vi "EventsDemo-Empty.vi"() -> ()   [LabVIEW 2014]
doc: "Use this template to build a user interface event handler design pattern. Use this pattern for dialog boxes and other user interfaces. You also can create and execute user-defined events that the VI can handle the same way as user interface events."
panel:
  in  "stop":bool
  out "Blink":bool
  in  "Blink Rate (ms)":i32
  in  "Value In":dbl(slide) scale=0.0..10.0
  out "Last Button":cluster{"1":bool, "2":bool, "3":bool}
  out "2 x Value":dbl
  in  "Button 3":bool
  in  "Button 2":bool
  in  "Button 1":bool
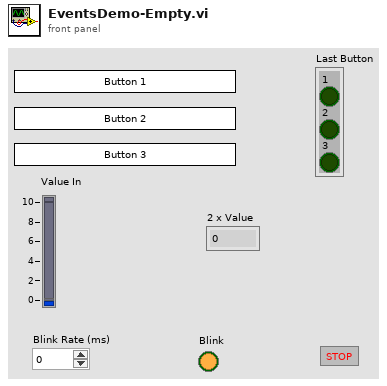
[diagram p1: front panel]
types:
  T1 = cluster{"Button 1":bool, "Button 2":bool, "Button 3":bool}
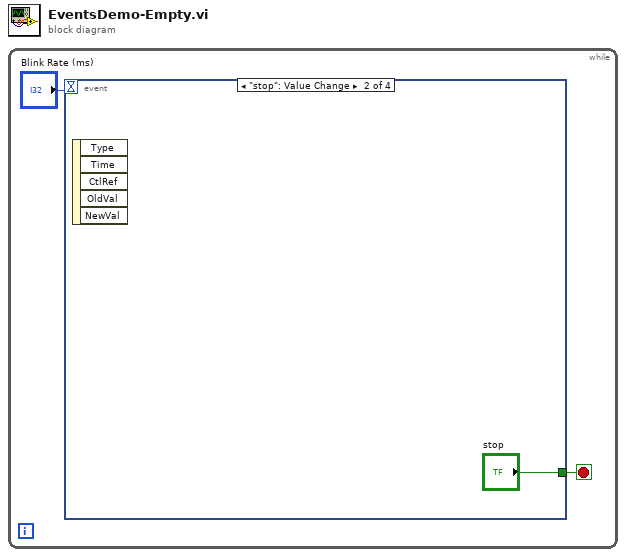
[diagram p0: block diagram]
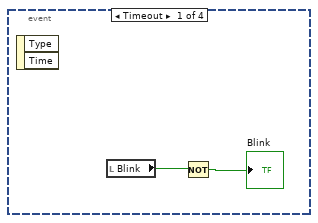
[diagram p2: hidden frame]
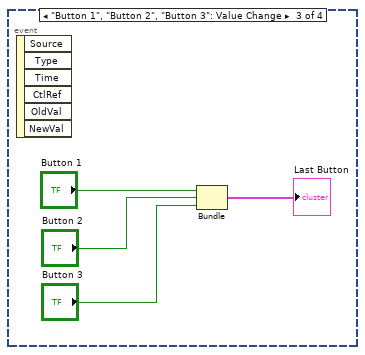
[diagram p3: hidden frame]
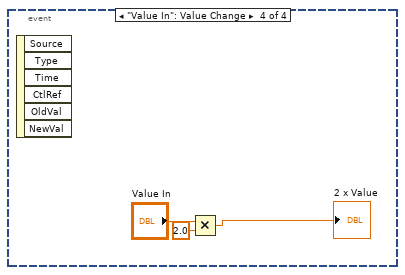
[diagram p4: hidden frame]
diagram:
  n1 = while {
    stop <- w2 stop-if-true
    n2 = event shown="[1] \"stop\": Value Change" {
      selector: _ -> [_ _ _ _]
      dyn-events: _ -> [_ _ _ _]
      timeout: "Blink Rate (ms)" -> [_ _ _ _]
      tunnel: [_ "stop" _ _] -> w2
      event Timeout {
        n3 = event-data() -> ()  [unwired: 1 in, 2 out]
        n4 = local read "Blink"() -> (w4:bool)
        n5 = Not(x=w4) -> (.not. x?=→"Blink":bool)
      }
      event "stop": Value Change {
        n6 = event-data() -> ()  [unwired: 1 in, 5 out]
      }
      event "Button 1", "Button 2", "Button 3": Value Change {
        n7 = event-data() -> ()  [unwired: 1 in, 6 out]
        n8 = Bundle("Button 1"="Button 1", "Button 2"="Button 2", "Button 3"="Button 3") -> (→"Last Button":T1)  [unwired: 1 in]
      }
      event "Value In": Value Change {
        n9 = event-data() -> ()  [unwired: 1 in, 6 out]
        n10 = Multiply(x="Value In", y=2.0) -> (x*y=→"2 x Value":dbl)
      }
    }
  }
